vi "toJSON.vi"(8 "error in (no error)":errorcluster, 11 "tBSONDocumentElement in":refnum<class "tBSONDocumentElement.lvclass">) -> (0 "error out":errorcluster, 2 "JSON":string, 3 "tBSONDocumentElement out":refnum<class "tBSONDocumentElement.lvclass">)   [LabVIEW 2013, in "BSON.lvlib" / "tBSONDocumentElement.lvclass"]
uses:
  tBSONDocumentElement.lvclass
  tBSONElement/tBSONElement.lvclass
  tBSONDocument/tBSONDocument.lvclass
  getValue.vi
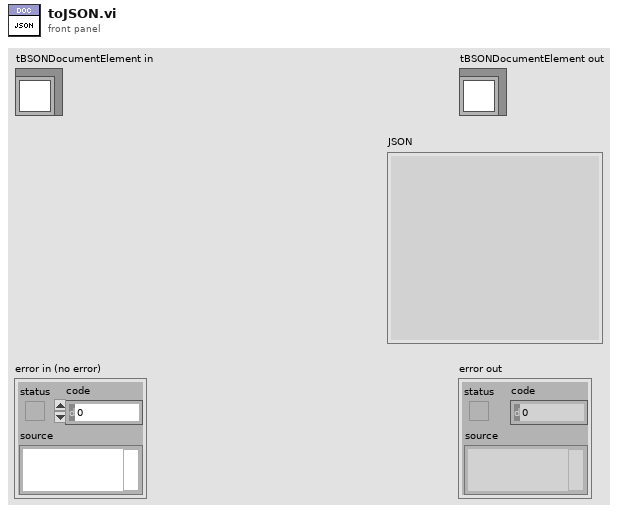
[diagram p1: front panel]
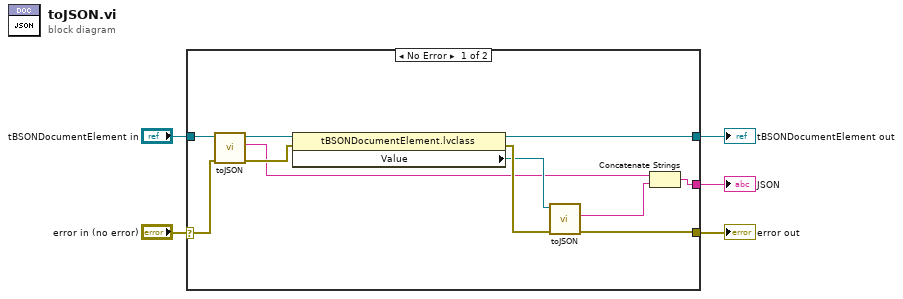
[diagram p0: block diagram]
diagram:
  n1 = case shown="No Error" "error in (no error)" {
    selector: "error in (no error)" -> [w15 w17]
    tunnel: [w7 w17] -> w5
    tunnel: [w6 _] -> w4
    tunnel: [w10 w18] -> w3
    tunnel: "tBSONDocumentElement in" -> [w16 w18]
    frame No Error {
      n2 = call-parent "toJSON.vi"("error in (no error)"=w15, "tBSONElement in"=w16) -> ("error out"=w13:errorcluster, "JSON"=w9:string, "tBSONElement out"=w14:refnum<class "tBSONDocumentElement.lvclass">)  [unwired: 7 in]
      n3 = property class="tBSONDocumentElement.lvclass"(reference=w14, error in=w13) -> (reference out=w10:refnum<class "tBSONDocumentElement.lvclass">, error out=w12:errorcluster, "Value"=w11:refnum<class "tBSONDocument.lvclass">)
      n4 = call-dynamic "toJSON.vi"("error in (no error)"=w12, "tBSONDocument in"=w11) -> ("error out"=w7:errorcluster, "JSON"=w8:string)  [unwired: 7 in, 1 out]
      n5 = Concatenate Strings(w9, w8) -> (w6:string)
    }
    frame Error {
    }
  }
  "error out" <- w5
  "tBSONDocumentElement out" <- w3
  "JSON" <- w4
